vi "Main.vi"(8 "error in (no error)":errorcluster, 11 "ModuleAdmin":refnum<class "ModuleAdmin.lvclass">) -> ()   [LabVIEW 2014, in "ScopeModule.lvlib"]
uses:
  ScopeModule.lvlib
  <userlib>/NIST/ModuleAdminLib/ModuleAdmin/ModuleAdmin.lvclass
  ScopePlugins/ScopePluginBaseClass/ScopePluginsBase.lvclass/ScopePluginsBase.ctl
  PublicAPI/Arguments/Requests/clStopArgument.ctl
  ScopePlugins/ScopePluginBaseClass/ScopePluginsBase.lvclass
  <userlib>/NIST/ModuleAdminLib/ModuleAdmin/ModuleAdmin.lvclass/ModuleAdmin.ctl
  <userlib>/NIST/BaseClasses/BasePlugin_class/BasePlugin.lvclass/BasePlugin.ctl
  ScopePlugins/InfiniiumClass/Typedefs/ExtAcquisition.ctl
  ScopePlugins/TypeDefs/InitOptions.ctl
  <vilib>/Utility/error.llb/DialogType.ctl
  ScopePlugins/ScopePluginBaseClass/Accessors/Read ModuleID.vi
  ScopePlugins/ScopePluginBaseClass/Accessors/Read Acquisition.vi
  ScopePlugins/ScopePluginBaseClass/Accessors/Read Channels.vi
  <userlib>/NIST/ModuleAdminLib/ModuleAdmin/Accessors/Read ShowPanel_.vi
  ScopePlugins/ScopePluginBaseClass/Accessors/Write ModuleID.vi
  <userlib>/NIST/ModuleAdminLib/ModuleAdmin/Accessors/Write ShowPanel_.vi
  <userlib>/NIST/BaseClasses/BasePlugin_class/Accessors/Read PluginIniFilePath.vi
  <userlib>/NIST/ModuleAdminLib/ModuleAdmin/Accessors/Read CloneRegRef.vi
  <vilib>/Utility/error.llb/Error Cluster From Error Code.vi
  <vilib>/ErrorRing/Error Ring.xnode
  <userlib>/NIST/ModuleAdminLib/CloneRegistration/CloneRegistration.lvclass
  <userlib>/NIST/ModuleAdminLib/ModuleAdmin.lvlib
  <userlib>/NIST/BaseClasses/Object_class/BaseObject.lvclass
  ScopePlugins/InfiniiumClass/Infiniium.lvclass
  ScopePlugins/ScopePlugins.lvlib
panel:
  out "error out":errorcluster
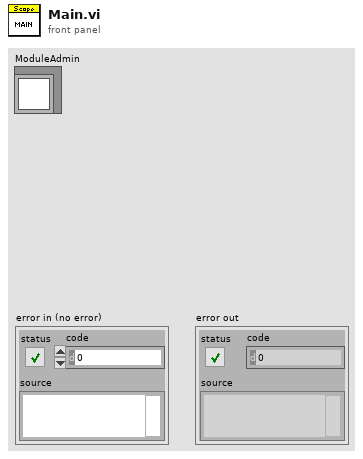
[diagram p1: front panel]
types:
  T1 = typedef "ScopeModule.lvlib/clRequestEvents.ctl" = cluster{"StopRequest":refnum<user-event>, "PathToINI":refnum<user-event>, " LoadPlugin":refnum<user-event>, "ShowPanel":refnum<user-event>, "Abort":refnum<user-event>, "SetAcquisition":refnum<user-event>, "SetChannel":refnum<user-event>, "SetTrigger":refnum<user-event>, "GetAcquisition":refnum<user-event>, "GetChannel":refnum<user-event>, "GetTrigger":refnum<user-event>, "FetchWaveform":refnum<user-event>, "InitAcquisition":refnum<user-event>, "ReadWaveform":refnum<user-event>, "GetHandle":refnum<user-event>, "SetHandle":refnum<user-event>, "GetModel":refnum<user-event>, "SetModel":refnum<user-event>, "ConfigAquisition":refnum<user-event>, "ConfigChannels":refnum<user-event>, "ConfigTrigger":refnum<user-event>, "Initialize":refnum<user-event>, "SetExtAcquisition":refnum<user-event>, "StopAcquisition":refnum<user-event>, "PrefDlg":refnum<user-event>, "Close":refnum<user-event>}
  T2 = typedef "ScopeModule.lvlib/clBroadcastEvents.ctl" = cluster{"DidInit":refnum<user-event>, "StatusUpdate":refnum<user-event>, "ErrorReport":refnum<user-event>, "DidStop":refnum<user-event>, "PathToINI":refnum<user-event>, "Handle":refnum<user-event>, "Model":refnum<user-event>, "Channels":refnum<user-event>, "Acquisition":refnum<user-event>, "Trigger":refnum<user-event>, "ExtAcquisition":refnum<user-event>, "Waveform":refnum<user-event>}
  T3 = typedef "ScopeModule.lvlib/clStopArgument.ctl" = cluster{"Exit via Stop Module Req?":bool, "Wait for Module to stop?":bool, "ModuleAdmin":refnum<class "ModuleAdmin.lvclass">}
  T4 = enum32{"Invalid", "Standard", "Closed", "Hidden", "Minimized", "Maximized"}
  T5 = typedef "ScopePlugins.lvlib/Infiniium.lvclass/ExtAcquisition.ctl" = cluster{"SamplingMode ":enum16{"Real Time", "Equivalent Time", "Segment", "Real Time Peak Detect", "Real Time High Resolution", "Peak Detect Segment", "High Resolution Segment"}, "Interpolation":enum16{"No Interpolation", "sin(x)/x", "linear", "1 Point sin(x)/x", "2 Point sin(x)/x", "4 Point sin(x)/x", "8 Point sin(x)/x", "16 Point sin(x)/x"}, "NumAverages":i32, "EnableAveraging":bool, "Resolution":enum16{"Auto", "Bits 9", "Bits 10", "Bits 11", "Bits 12"}}
  T6 = typedef "ScopePlugins.lvlib/InitOptions.ctl" = cluster{"Reset":bool, "IdQuery":bool}
  T7 = typedef "ScopePlugins.lvlib/Acquisition.ctl" = cluster{"StartTime":dbl, "Type":enum16{"Normal", "PeakDetect", "HighRes", "Envelope", "Average"}, "NumPointsMin":i32, "RecordLength":i32, "SampleRate":dbl, "TimePerRecord":dbl, "SamplingMode ":enum16{"Real Time", "Equivalent Time", "Segment", "Real Time Peak Detect", "Real Time High Resolution", "Peak Detect Segment", "High Resolution Segment"}, "Interpolation":enum16{"No Interpolation", "sin(x)/x", "linear", "1 Point sin(x)/x", "2 Point sin(x)/x", "4 Point sin(x)/x", "8 Point sin(x)/x", "16 Point sin(x)/x"}, "NumAverages":i32, "Resolution":enum16{"Auto", "Bits 9", "Bits 10", "Bits 11", "Bits 12"}, "EnableAveraging":bool, "Continuous":bool}
  T8 = typedef "ScopePlugins.lvlib/Channels.ctl" = cluster{"Count":i32, "ChannelArray":T9[]}
  T9 = typedef "ScopePlugins.lvlib/Channel.ctl" = cluster{"Enabled":bool, "Name":string, "InputImpedance":dbl, "InputFreqMax":dbl, "ProbeAttn":dbl, "Coupling":enum16{"AC", "DC", "GND"}, "Offset":dbl, "Range":dbl, "Handle":string, "Connected":bool}
  T10 = typedef "ScopePlugins.lvlib/Waveform.ctl" = cluster{"initial x":dbl, "x increment":dbl, "waveform array":dbl[]}
  T11 = typedef "DialogType.ctl" = u16
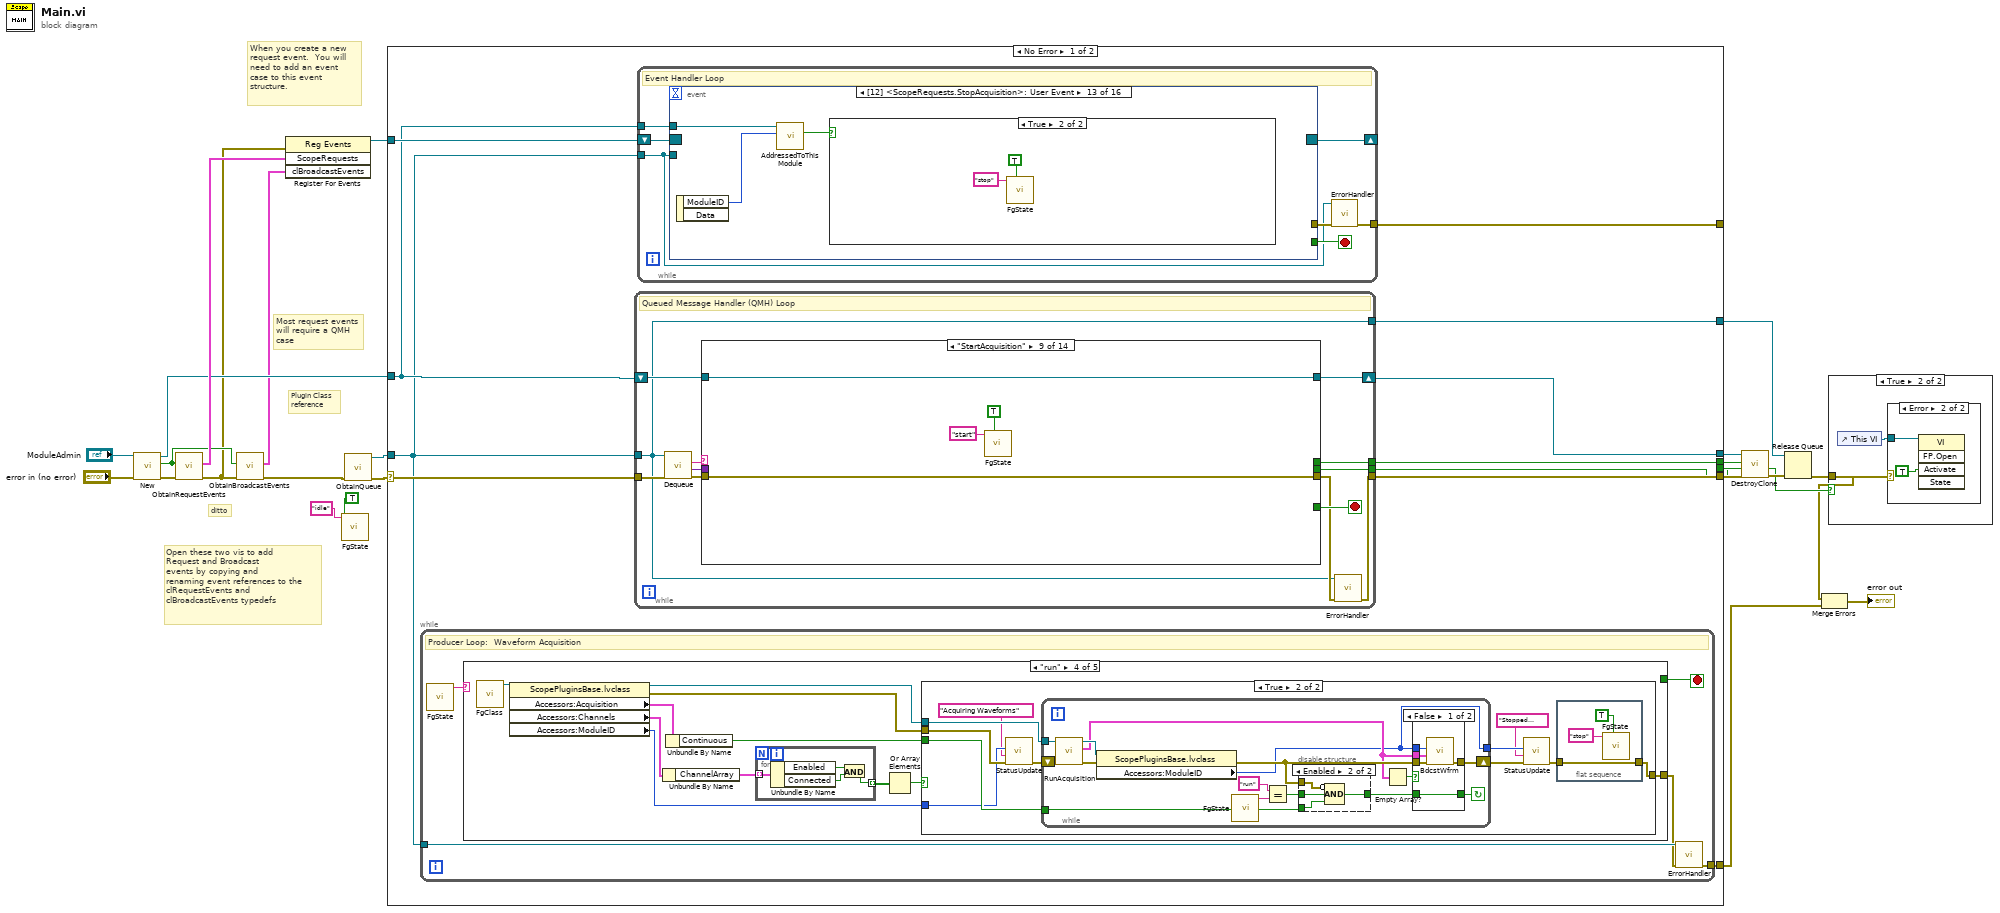
[diagram p0: block diagram]
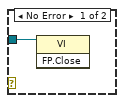
[diagram p3: hidden frame]
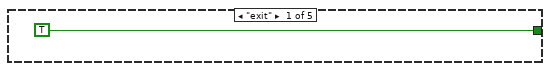
[diagram p4: hidden frame]
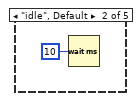
[diagram p5: hidden frame]
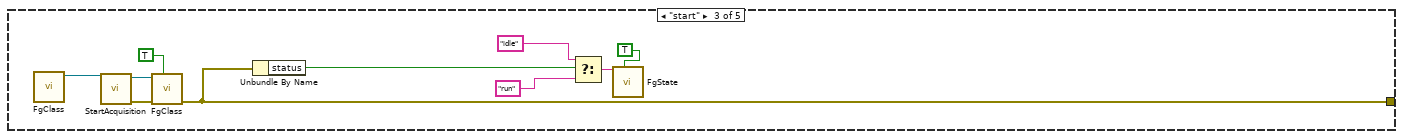
[diagram p6: hidden frame]
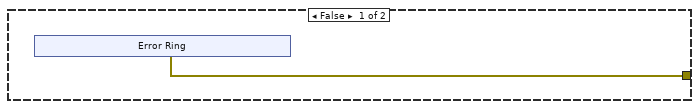
[diagram p7: hidden frame]
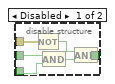
[diagram p8: hidden frame]
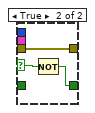
[diagram p9: hidden frame]
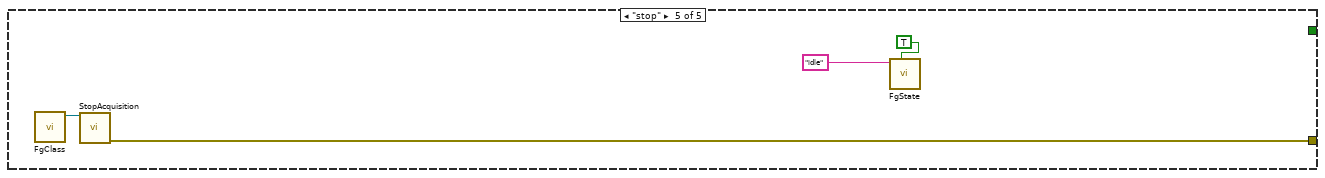
[diagram p10: hidden frame]
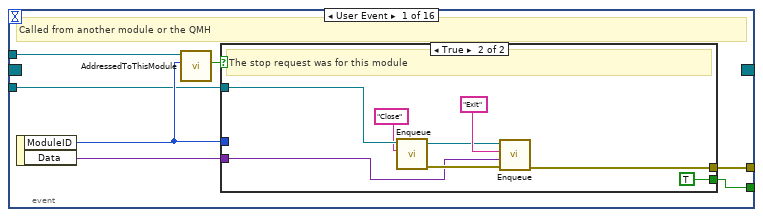
[diagram p11: hidden frame]
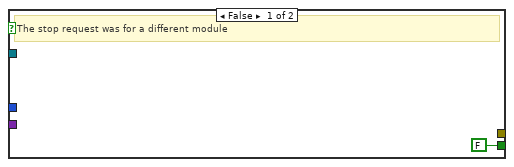
[diagram p12: hidden frame]
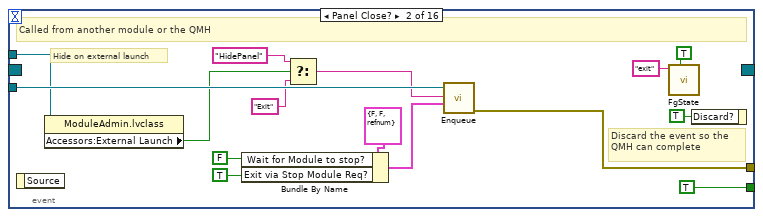
[diagram p13: hidden frame]
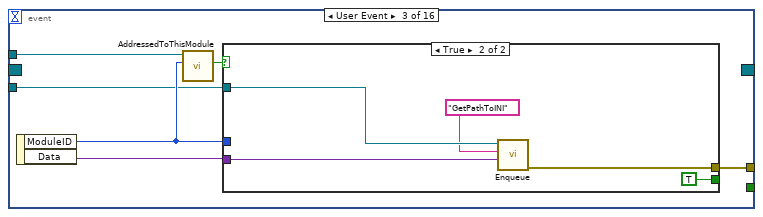
[diagram p14: hidden frame]
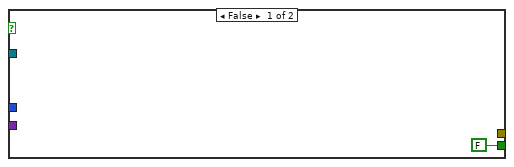
[diagram p15: hidden frame]
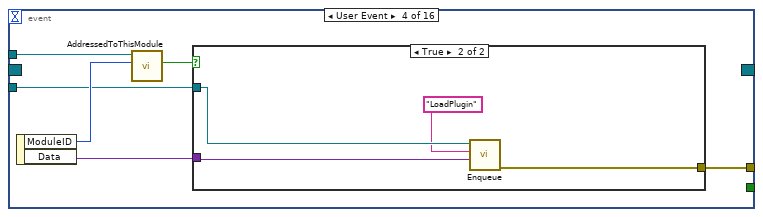
[diagram p16: hidden frame]
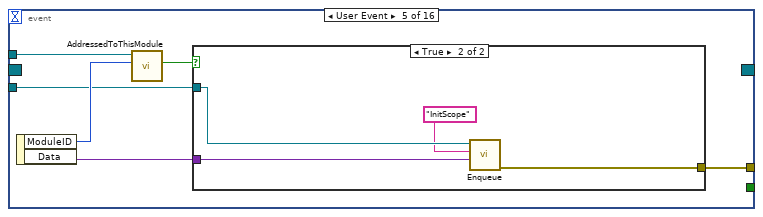
[diagram p18: hidden frame]
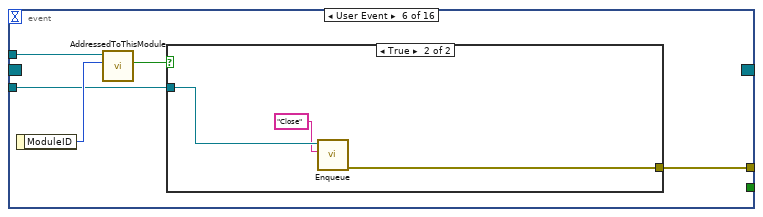
[diagram p20: hidden frame]
diagram:
  # "Plugin Class\nreference"
  # "Open these two vis to add\nRequest and Broadcast \nevents by copying and \nrenaming event references to the \nclRequestEvents and \nclBroadcastEvents typedefs"
  # "ditto"
  # "Most request events\nwill require a QMH\ncase"
  # "When you create a new request event.  You will need to add an event case to this event structure."
  n1 = call <userlib>:"New.vi"("error in (no error)"="error in (no error)", "ModuleAdmin"="ModuleAdmin") -> ("error out"=w22:errorcluster, "First?"=w15:bool, "ModuleAdmin"=w18:refnum<class "ModuleAdmin.lvclass">)  [unwired: 6 in, 1 out]
  n2 = call "ObtainRequestEvents.vi"("error in (no error)"=w22, "CreateNew (F)"=w15) -> ("error out"=w14:errorcluster, "ScopeRequests"=w21:T1)  [unwired: 8 in]
  n3 = call "ObtainBroadcastEvents.vi"("error in (no error)"=w14, "CreateNew? (F)"=w15) -> ("error out"=w16:errorcluster, "clBroadcastEvents"=w13:T2)  [unwired: 8 in]
  n4 = register-events(error in=w14, w21, w13) -> (reference out=w12:refnum<event-registration>)  [unwired: 1 in, 1 out]
  n5 = call "FgState.vi"("Set (F)"=TRUE, "State In"="idle") -> ()  [unwired: 9 in, 1 out]
  n6 = call "ObtainQueue.vi"("error in (no error)"=w16) -> ("error out"=w20:errorcluster, "MessageQueue"=w19:refnum<queue>)  [unwired: 9 in]
  n7 = case shown="No Error" w20 {
    selector: w20 -> [w35 w535]
    tunnel: w19 -> [w26 w531]
    tunnel: w18 -> [w31 w532]
    tunnel: [w34 w533] -> w11
    tunnel: [w33 w531] -> w17
    tunnel: w12 -> [w32 _]
    tunnel: [w30 w530] -> w9
    tunnel: [w29 _] -> w8
    tunnel: [w28 _] -> w7
    tunnel: [w27 _] -> _
    tunnel: [w25 _] -> w1
    frame No Error {
      n8 = while {
        tunnel: w26 -> [w38]
        tunnel: [w36] -> w25
        stop <- w39 stop-if-true
        # "Producer Loop:  Waveform Acquisition"
        n9 = call "FgState.vi"() -> ("State Out"=w40:string)  [unwired: 11 in]
        n10 = case shown="\"run\"" w40 {
          tunnel: [TRUE _ _ _ _] -> w39
          tunnel: [_ _ w48 w61 w120] -> w37
          frame "exit" {
          }
          frame "idle", Default {
            n11 = Wait (ms)(milliseconds to wait=u32 10) -> ()  [unwired: 1 out]
          }
          frame "start" {
            n12 = call "FgClass.vi"() -> ("Class Out"=w51:refnum<class "ScopePluginsBase.lvclass">)  [unwired: 11 in]
            n13 = call-dynamic "StartAcquisition.vi"("ScopePluginsBase in"=w51) -> ("error out"=w48:errorcluster, "ScopePluginsBase out"=w50:refnum<class "ScopePluginsBase.lvclass">)  [unwired: 9 in]
            n14 = call "FgClass.vi"("Set (F)"=TRUE, "Class In"=w50) -> ()  [unwired: 9 in, 1 out]
            n15 = Unbundle By Name(w48) -> ("status"=w46:bool)
            n16 = Select(t="idle" ("State In"), s=w46, f="run") -> (s? t:f=w44:string)
            n17 = call "FgState.vi"("Set (F)"=TRUE, "State In"=w44) -> ()  [unwired: 9 in, 1 out]
          }
          frame "run" {
            n18 = call "FgClass.vi"() -> ("Class Out"=w62:refnum<class "ScopePluginsBase.lvclass">)  [unwired: 11 in]
            n19 = property class="ScopePluginsBase.lvclass"(reference=w62) -> (reference out=w60:refnum<class "ScopePluginsBase.lvclass">, error out=w58:errorcluster, "Accessors:Acquisition"=w53:T7, "Accessors:Channels"=w54:T8, "Accessors:ModuleID"=w52:i32)  [unwired: 1 in]
            n20 = Unbundle By Name(w54) -> ("ChannelArray"=w57:T9[])
            n21 = Unbundle By Name(w53) -> ("Continuous"=w59:bool)
            n22 = for {
              tunnel: w57 -> [w66] mode=indexing
              tunnel: [w63] -> w56 mode=indexing
              n23 = Unbundle By Name(w66) -> ("Enabled"=w65:bool, "Connected"=w64:bool)
              n24 = And(x=w65, y=w64) -> (x .and. y?=w63:bool)
            }
            n25 = Or Array Elements(Boolean array=w56) -> (logical OR=w55:bool)
            n26 = case shown="True" w55 {
              tunnel: [w67 w81] -> w61
              tunnel: w60 -> [_ w83]
              tunnel: w59 -> [_ w82]
              tunnel: w58 -> [_ w80]
              tunnel: w52 -> [_ w78]
              frame False {
                n27 = xnode "Error Ring"() -> ("error out"=w67:errorcluster)
              }
              frame True {
                n28 = call "StatusUpdate.vi"("error in (no error)"=w80, "Status"="Acquiring Waveforms", "ModuleID"=w78) -> ("error out"=w79:errorcluster)  [unwired: 8 in]
                n29 = while {
                  tunnel: w83 -> [w98]
                  tunnel: w82 -> [w97]
                  shift-right: [w95] -> w76
                  shift-left: w79 -> [w96]
                  tunnel: [w84] -> w74
                  stop <- w85 continue-if-true
                  n30 = call-dynamic "RunAcquisition.vi"("error in (no error)"=w96, "ScopePluginsBase in"=w98) -> ("error out"=w90:errorcluster, "Waveforms"=w88:T10[], "ScopePluginsBase out"=w91:refnum<class "ScopePluginsBase.lvclass">)  [unwired: 7 in]
                  n31 = property class="ScopePluginsBase.lvclass"(reference=w91, error in=w90) -> (error out=w89:errorcluster, "Accessors:ModuleID"=w84:i32)  [unwired: 1 out]
                  n32 = call "FgState.vi"() -> ("State Out"=w94:string)  [unwired: 11 in]
                  n33 = Equal?(x="run", y=w94) -> (x = y?=w92:bool)
                  n34 = disable-structure shown="Enabled" {
                    disable-tunnel: w97 -> [w104 w108]
                    disable-tunnel: w92 -> [w103 w106]
                    disable-tunnel: w89 -> [w100 w107]
                    disable-tunnel: [w99 w105] -> w86
                    frame Disabled {
                      n35 = Not(x=w100) -> (.not. x?=w101:bool)
                      n36 = And(x=w103, y=w104) -> (x .and. y?=w102:bool)
                      n37 = And(x=w101, y=w102) -> (x .and. y?=w99:bool)
                    }
                    frame Enabled {
                      n38 = Compound Arithmetic op=AND(invert w107, w106, w108) -> (w105:bool)
                    }
                  }
                  n39 = Empty Array?(array=w88) -> (empty?=w87:bool)
                  n40 = case shown="False" w87 {
                    selector: w87 -> [_ w115]
                    tunnel: [w113 w116] -> w95
                    tunnel: w88 -> [w112 _]
                    tunnel: w84 -> [w111 _]
                    tunnel: w89 -> [w110 w116]
                    tunnel: w86 -> [w109 _]
                    tunnel: [w109 w114] -> w85
                    frame False {
                      n41 = call "BdcstWfrm.vi"("error in (no error)"=w110, "Waveforms"=w112, "ModuleID"=w111) -> ("error out"=w113:errorcluster)  [unwired: 8 in]
                    }
                    frame True {
                      n42 = Not(x=w115) -> (.not. x?=w114:bool)
                    }
                  }
                }
                n43 = call "StatusUpdate.vi"("error in (no error)"=w76, "Status"="Stopped Acquisition", "ModuleID"=w74) -> ("error out"=w75:errorcluster)  [unwired: 8 in]
                n44 = flat-sequence {
                  tunnel: w75 -> [w117]
                  tunnel: [w117] -> w81
                  frame #0 {
                    n45 = call "FgState.vi"("Set (F)"=TRUE, "State In"="stop") -> ()  [unwired: 9 in, 1 out]
                  }
                }
              }
            }
          }
          frame "stop" {
            n46 = call "FgClass.vi"() -> ("Class Out"=w121:refnum<class "ScopePluginsBase.lvclass">)  [unwired: 11 in]
            n47 = call-dynamic "StopAcquisition.vi"("ScopePluginsBase in"=w121) -> ("error out"=w120:errorcluster)  [unwired: 9 in, 1 out]
            n48 = call "FgState.vi"("Set (F)"=TRUE, "State In"="idle") -> ()  [unwired: 9 in, 1 out]
          }
        }
        n49 = call "ErrorHandler.vi"("error in (no error)"=w37, "MessageQueue"=w38) -> ("error out"=w36:errorcluster)  [unwired: 8 in, 1 out]
      }
      n50 = while {
        tunnel: w26 -> [w293]
        tunnel: w35 -> [w302]
        tunnel: [w295] -> w34
        tunnel: [w293] -> w33
        tunnel: [w297] -> w29
        tunnel: [w296] -> w28
        shift-right: [w292] -> w30
        shift-left: w31 -> [w298]
        stop <- w303 stop-if-true
        # "Queued Message Handler (QMH) Loop"
        n51 = call "Dequeue.vi"("error in (no error)"=w302, "MessageQueue"=w293) -> ("error out"=w301:errorcluster, "Message Data"=w299:variant, "Message"=w300:string)  [unwired: 6 in, 1 out]
        n52 = case shown="\"StartAcquisition\"" w300 {
          selector: w300 -> [_ _ _ _ _ _ _ _ _ _ _ _ _ w516]
          tunnel: [_ _ _ _ _ _ _ _ _ _ _ TRUE _ _] -> w303
          tunnel: w298 -> [w326 w342 w351 w357 w404 w419 w432 w446 w453 w465 w474 w490 w504 w519]
          tunnel: [w315 w335 w352 w358 w405 w415 w430 w445 w456 w463 w475 w497 w501 w515] -> w294
          tunnel: w301 -> [_ w345 w349 w367 w409 w418 w433 w447 w456 w471 w483 w489 w505 _]
          tunnel: w299 -> [_ w344 _ w369 w410 _ _ _ _ w472 w482 w493 _ _]
          tunnel: [_ _ _ _ _ _ _ _ _ _ _ w495 _ _] -> w297
          tunnel: [_ _ _ _ _ _ _ _ _ _ _ w494 _ _] -> w296
          tunnel: [w308 w341 w347 w354 w404 w417 w429 w443 w453 w462 w473 w490 w500 w513] -> w292
          frame "Initialize" {
            # "Initialize is always called after ObtainQueue.vi is run"
            n53 = property class="ModuleAdmin.lvclass"(reference=w326) -> (reference out=w313:refnum<class "ModuleAdmin.lvclass">, error out=w323:errorcluster, "Accessors:Module ID"=w304:i32, "Accessors:ShowPanel_"=w311:bool, "Accessors:External Launch"=w310:bool, "Accessors:ModuleName"=w312:string)  [unwired: 1 in]
            n54 = property class="ScopePluginsBase.lvclass"(reference=refnum<class "ScopePluginsBase.lvclass"> refnum ("MyPlugins.lvlib:MyPluginsBase.lvclass"), "Accessors:ModuleID"=w304) -> (reference out=w305:refnum<class "ScopePluginsBase.lvclass">)  [unwired: 1 in, 1 out]
            n55 = Compound Arithmetic op=OR(w311, invert w310) -> (w309:bool)
            n56 = Select(t=T4."Standard" ("Front Panel Window:State"), s=w309, f=T4."Hidden" ("Front Panel Window:State")) -> (s? t:f=w319:T4)
            n57 = call "FgClass.vi"("Set (F)"=TRUE, "Class In"=w305) -> ()  [unwired: 9 in, 1 out]
            n58 = invoke class="VI" method="FP.Open"(error in=w323, "State"=w319) -> (error out=w322:errorcluster)  [unwired: 3 in, 4 out]
            n59 = call <userlib>:"ModuleName.vi"("Name"=w312, "ModuleID"=w304) -> ("ModuleName"=w318:string)  [unwired: 9 in]
            n60 = property class="VI"(error in=w322, "Front Panel.Title"=w318) -> (reference out=w325:refnum<vi>, error out=w324:errorcluster)  [unwired: 1 in]
            n61 = invoke class="VI" method="FP.Center"(reference=w325, error in=w324) -> (error out=w314:errorcluster)  [unwired: 1 in, 2 out]
            n62 = case shown="True" w310 {
              tunnel: [w327 w333] -> w316
              tunnel: [w328 w330] -> w308
              tunnel: w314 -> [w327 w332]
              tunnel: w313 -> [w328 w329]
              frame False {
              }
              frame True {
                n63 = call <userlib>:"WaitOnModuleSync.vi"("error in (no error)"=w332, "ModuleAdmin"=w329) -> ("error out"=w334:errorcluster, "ModuleAdmin"=w331:refnum<class "ModuleAdmin.lvclass">)  [unwired: 8 in]
                n64 = call <userlib>:"WaitOnEventSync.vi"("error in (no error)"=w334, "ModuleAdmin"=w331) -> ("error out"=w333:errorcluster, "ModuleAdmin"=w330:refnum<class "ModuleAdmin.lvclass">)  [unwired: 8 in]
              }
            }
            n65 = call "DidInit.vi"("Init?"=TRUE, "error in (no error)"=w316, "ModuleAdmin"=w308) -> ("error out"=w315:errorcluster)  [unwired: 8 in]
          }
          frame "ShowPanel" {
            n66 = Variant To Data(error in=w345, type=TRUE, Variant=w344) -> (data=w337:bool, error out=w340:errorcluster)
            n67 = Select(t=T4."Standard" ("Front Panel Window:State"), s=w337, f=T4."Hidden" ("Front Panel Window:State")) -> (s? t:f=w336:T4)
            n68 = property class="VI"(error in=w340, "FP.State"=w336) -> (error out=w335:errorcluster)  [unwired: 1 in, 1 out]
            n69 = property class="ModuleAdmin.lvclass"(reference=w342, "Accessors:ShowPanel_"=w337) -> (reference out=w341:refnum<class "ModuleAdmin.lvclass">)  [unwired: 1 in, 1 out]
          }
          frame "GetPathToINI" {
            n70 = call "FgClass.vi"() -> ("Class Out"=w346:refnum<class "ScopePluginsBase.lvclass">)  [unwired: 11 in]
            n71 = property class="ScopePluginsBase.lvclass"(reference=w346, error in=w349) -> (error out=w348:errorcluster, "Accessors:PluginIniFilePath"=w350:path)  [unwired: 1 out]
            n72 = property class="ModuleAdmin.lvclass"(reference=w351) -> (reference out=w347:refnum<class "ModuleAdmin.lvclass">, "Accessors:Module ID"=w353:i32)  [unwired: 1 in, 1 out]
            n73 = call "PathToINIBroadcast.vi"("error in (no error)"=w348, "PathToINI"=w350, "ModuleID"=w353) -> ("error out"=w352:errorcluster)  [unwired: 8 in]
          }
          frame "LoadPlugin" {
            n74 = Variant To Data(error in=w367, type=path "", Variant=w369) -> (data=w355:path, error out=w366:errorcluster)
            n75 = disable-structure shown="Enabled" {
              disable-tunnel: [w372 w373] -> w356
              disable-tunnel: w355 -> [w370 w373]
              frame Disabled {
                n76 = Current VI's Path() -> (path=w371:path)
                n77 = Build Path(base path=w371, name or relative path=w370) -> (appended path=w372:path)
              }
              frame Enabled {
              }
            }
            n78 = call <userlib>:"GetPathToClass.vi"("error in (no error)"=w366, "configuration file path"=w356) -> ("error IO"=w362:errorcluster, "PathToClass"=w365:path)  [unwired: 8 in]
            n79 = Current VI's Path() -> (path=w364:path)
            n80 = Build Path(base path=w364, name or relative path=w365) -> (appended path=w363:path)
            n81 = call <vilib>:"Check if File or Folder Exists.vi"("error in (no error)"=w362, "path"=w363) -> ("error out"=w359:errorcluster, "file or folder exists?"=w361:bool, "dup path"=w360:path)  [unwired: 7 in]
            n82 = case shown="True" w361 {
              tunnel: w360 -> [w376 w392]
              tunnel: w359 -> [_ w400]
              tunnel: [w375 w395] -> w358
              tunnel: w357 -> [w374 w394]
              tunnel: w355 -> [_ w388]
              tunnel: [w374 w391] -> w354
              frame False {
                n83 = Path To String(path=w376) -> (string=w377:string)
                n84 = xnode "Error Ring"("parameter 0"=w377) -> ("error out"=w375:errorcluster)
              }
              frame True {
                n85 = call-dynamic "LoadClassFromFile.vi"("error in (no error)"=w400, "class path"=w392, "reference in"=refnum<class "ScopePluginsBase.lvclass"> refnum ("MyPlugins.lvlib:MyPluginsBase.lvclass")) -> ("error out"=w389:errorcluster, "reference out"=w390:refnum<class "ScopePluginsBase.lvclass">)  [unwired: 7 in]
                n86 = property class="ModuleAdmin.lvclass"(reference=w394) -> (reference out=w391:refnum<class "ModuleAdmin.lvclass">, "Accessors:Module ID"=w393:i32)  [unwired: 1 in, 1 out]
                n87 = call-dynamic "GetDefaultParams.vi"("error in (no error)"=w389, "config file path"=w388, "ScopeBase"=w390) -> ("error out"=w387:errorcluster, "ScopeBase"=w386:refnum<class "ScopePluginsBase.lvclass">)  [unwired: 6 in, 1 out]
                n88 = Path To String(path=w392) -> (string=w397:string)
                n89 = call "FgClass.vi"("Set (F)"=TRUE, "Class In"=w386) -> ()  [unwired: 9 in, 1 out]
                n90 = Format Into String(format string="Plugin %s loaded ", w397) -> (resulting string=w396:string)  [unwired: 2 in, 1 out]
                n91 = call "StatusUpdate.vi"("error in (no error)"=w387, "Status"=w396, "ModuleID"=w393) -> ("error out"=w395:errorcluster)  [unwired: 8 in]
              }
            }
          }
          frame "SetExtAquisition" {
            n92 = Variant To Data(error in=w409, type=T5 {"SamplingMode "=enum."Real Time", "Interpolation"=enum."No Interpolation", "NumAverages"=8, "EnableAveraging"=FALSE, "Resolution"=enum."Auto"} ("ExtAcquisition"), Variant=w410) -> (data=w406:T5, error out=w407:errorcluster)
            n93 = call "FgClass.vi"() -> ("Class Out"=w403:refnum<class "ScopePluginsBase.lvclass">)  [unwired: 11 in]
            n94 = call-dynamic "SetExtAcquisition.vi"("error in (no error)"=w407, "ExtAcquisition"=w406, "ScopePluginsBase in"=w403) -> ("error out"=w405:errorcluster, "ScopePluginsBase out"=w402:refnum<class "ScopePluginsBase.lvclass">)  [unwired: 7 in]
            n95 = call "FgClass.vi"("Set (F)"=TRUE, "Class In"=w402) -> ()  [unwired: 9 in, 1 out]
          }
          frame "ConfigAcquisition" {
            n96 = call "FgClass.vi"() -> ("Class Out"=w413:refnum<class "ScopePluginsBase.lvclass">)  [unwired: 11 in]
            n97 = call-dynamic "ConfigureAcquisition.vi"("error in (no error)"=w418, "ScopePluginsBase in"=w413) -> ("error out"=w416:errorcluster, "ScopePluginsBase out"=w412:refnum<class "ScopePluginsBase.lvclass">)  [unwired: 8 in]
            n98 = call "FgClass.vi"("Set (F)"=TRUE, "Class In"=w412) -> ()  [unwired: 9 in, 1 out]
            n99 = property class="ModuleAdmin.lvclass"(reference=w419) -> (reference out=w417:refnum<class "ModuleAdmin.lvclass">, "Accessors:Module ID"=w414:i32)  [unwired: 1 in, 1 out]
            n100 = case shown="No Error" w416 {
              selector: w416 -> [w423 w424]
              tunnel: [w422 w424] -> w415
              tunnel: w414 -> [w421 _]
              frame No Error {
                n101 = call "StatusUpdate.vi"("error in (no error)"=w423, "Status"="Acquisition Configured", "ModuleID"=w421) -> ("error out"=w422:errorcluster)  [unwired: 8 in]
              }
              frame Error {
              }
            }
          }
          frame "ConfigChannels" {
            n102 = call "FgClass.vi"() -> ("Class Out"=w427:refnum<class "ScopePluginsBase.lvclass">)  [unwired: 11 in]
            n103 = call-dynamic "ConfigureChannels.vi"("error in (no error)"=w433, "ScopePluginsBase in"=w427) -> ("error out"=w431:errorcluster, "ScopePluginsBase out"=w426:refnum<class "ScopePluginsBase.lvclass">)  [unwired: 8 in]
            n104 = call "FgClass.vi"("Set (F)"=TRUE, "Class In"=w426) -> ()  [unwired: 9 in, 1 out]
            n105 = property class="ModuleAdmin.lvclass"(reference=w432) -> (reference out=w429:refnum<class "ModuleAdmin.lvclass">, "Accessors:Module ID"=w428:i32)  [unwired: 1 in, 1 out]
            n106 = case shown="No Error" w431 {
              selector: w431 -> [w437 w438]
              tunnel: [w436 w438] -> w430
              tunnel: w428 -> [w435 _]
              frame No Error {
                n107 = call "StatusUpdate.vi"("error in (no error)"=w437, "Status"="Channels Configured", "ModuleID"=w435) -> ("error out"=w436:errorcluster)  [unwired: 8 in]
              }
              frame Error {
              }
            }
          }
          frame "ConfigTrigger" {
            n108 = call "FgClass.vi"() -> ("Class Out"=w441:refnum<class "ScopePluginsBase.lvclass">)  [unwired: 11 in]
            n109 = call-dynamic "ConfigureTrigger.vi"("error in (no error)"=w447, "ScopePluginsBase in"=w441) -> ("error out"=w444:errorcluster, "ScopePluginsBase out"=w440:refnum<class "ScopePluginsBase.lvclass">)  [unwired: 8 in]
            n110 = call "FgClass.vi"("Set (F)"=TRUE, "Class In"=w440) -> ()  [unwired: 9 in, 1 out]
            n111 = property class="ModuleAdmin.lvclass"(reference=w446) -> (reference out=w443:refnum<class "ModuleAdmin.lvclass">, "Accessors:Module ID"=w442:i32)  [unwired: 1 in, 1 out]
            n112 = case shown="No Error" w444 {
              selector: w444 -> [w451 w452]
              tunnel: [w450 w452] -> w445
              tunnel: w442 -> [w449 _]
              frame No Error {
                n113 = call "StatusUpdate.vi"("error in (no error)"=w451, "Status"="Trigger Configured", "ModuleID"=w449) -> ("error out"=w450:errorcluster)  [unwired: 8 in]
              }
              frame Error {
              }
            }
          }
          frame "StartAcquisition" {
            n114 = call "FgState.vi"("Set (F)"=TRUE, "State In"="start") -> ()  [unwired: 9 in, 1 out]
          }
          frame "InitScope" {
            n115 = Variant To Data(error in=w471, type=T6 {"Reset"=FALSE, "IdQuery"=FALSE} ("InitOptions"), Variant=w472) -> (data=w469:T6, error out=w466:errorcluster)
            n116 = Unbundle By Name(w469) -> ("IdQuery"=w468:bool, "Reset"=w467:bool)
            n117 = call "FgClass.vi"() -> ("Class Out"=w459:refnum<class "ScopePluginsBase.lvclass">)  [unwired: 11 in]
            n118 = call-dynamic "Initialize.vi"("error in (no error)"=w466, "Reset (f)"=w467, "IdQuery (f)"=w468, "ScopePluginsBase in"=w459) -> ("error out"=w464:errorcluster, "ScopePluginsBase out"=w458:refnum<class "ScopePluginsBase.lvclass">)  [unwired: 6 in]
            n119 = call "FgClass.vi"("Set (F)"=TRUE, "Class In"=w458) -> ()  [unwired: 9 in, 1 out]
            n120 = property class="ModuleAdmin.lvclass"(reference=w465) -> (reference out=w462:refnum<class "ModuleAdmin.lvclass">, "Accessors:Module ID"=w461:i32)  [unwired: 1 in, 1 out]
            n121 = call "StatusUpdate.vi"("error in (no error)"=w464, "Status"="O'Scope hardware initialized", "ModuleID"=w461) -> ("error out"=w463:errorcluster)  [unwired: 8 in]
          }
          frame "Error" {
            n122 = property class="ModuleAdmin.lvclass"(reference=w474) -> (reference out=w473:refnum<class "ModuleAdmin.lvclass">, "Accessors:External Launch"=w478:bool, "Accessors:Module ID"=w476:i32)  [unwired: 1 in, 1 out]
            n123 = Variant To Data(error in=w483, type=errorcluster {"status"=FALSE, "code"=0, "source"=""} ("error constant"), Variant=w482) -> (data=w477:errorcluster, error out=w480:errorcluster)
            n124 = call "ReportError.vi"("error in (no error)"=w480, "ErrorReported"=w477, "ModuleID"=w476) -> ("error out"=w479:errorcluster)  [unwired: 8 in]
            n125 = case shown="True" w478 {
              tunnel: w479 -> [w487 w488]
              tunnel: w477 -> [w486 _]
              tunnel: [w485 w488] -> w475
              tunnel: w474 -> [w484 _]
              frame False {
                # "Todo:  Add an event to ask the user\nIf the module should stop or continue"
                # "Stand alone: now, force an exit"
                n126 = call <vilib>:"Simple Error Handler.vi"("error in (no error)"=w486) -> ()  [unwired: 4 in, 5 out]
                n127 = call "StopRequest.vi"("error in (no error)"=w487, "ModuleAdmin"=w484) -> ("error out"=w485:errorcluster)  [unwired: 8 in, 1 out]
              }
              frame True {
                # "Externally launched modules only broadcast the error msg"
              }
            }
          }
          frame "Exit" {
            # "Called by the StopRequest event handler case"
            n128 = control-ref of="This VI"() -> (w496:refnum<vi>)
            n129 = call "FgState.vi"("Set (F)"=TRUE, "State In"="exit") -> ()  [unwired: 9 in, 1 out]
            n130 = call "HandleExit.vi"("error in (no error)"=w489, "VI Refnum"=w496, "StopArgument"=w493, "ModuleAdmin"=w490) -> ("error out"=w497:errorcluster, "Exit via Stop Module Req?"=w494:bool, "WaitForStop?"=w495:bool)  [unwired: 5 in]
          }
          frame "Close" {
            n131 = call "FgClass.vi"() -> ("Class Out"=w507:refnum<class "ScopePluginsBase.lvclass">)  [unwired: 11 in]
            n132 = call-dynamic "Close.vi"("error in (no error)"=w505, "ScopePluginsBase in"=w507) -> ("error out"=w502:errorcluster, "ScopePluginsBase out"=w506:refnum<class "ScopePluginsBase.lvclass">)  [unwired: 8 in]
            n133 = call "FgClass.vi"("Set (F)"=TRUE, "Class In"=w506) -> ()  [unwired: 9 in, 1 out]
            n134 = property class="ModuleAdmin.lvclass"(reference=w504) -> (reference out=w500:refnum<class "ModuleAdmin.lvclass">, "Accessors:Module ID"=w499:i32)  [unwired: 1 in, 1 out]
            n135 = case shown="No Error" w502 {
              selector: w502 -> [w511 w512]
              tunnel: [w510 w512] -> w501
              tunnel: w499 -> [w509 _]
              frame No Error {
                n136 = call "StatusUpdate.vi"("error in (no error)"=w511, "Status"="O'Scope Disconnected", "ModuleID"=w509) -> ("error out"=w510:errorcluster)  [unwired: 8 in]
              }
              frame Error {
              }
            }
          }
          frame Default {
            # "Called only if a message was queued and no QMH case was created"
            n137 = property class="ModuleAdmin.lvclass"(reference=w519) -> (reference out=w513:refnum<class "ModuleAdmin.lvclass">, "Accessors:Module ID"=w518:i32, "Accessors:ModuleName"=w514:string)  [unwired: 1 in, 1 out]
            n138 = call <userlib>:"ModuleName.vi"("Name"=w514, "ModuleID"=w518) -> ("ModuleName"=w517:string)  [unwired: 9 in]
            n139 = xnode "Error Ring"("parameter 0"=w516, "parameter 1"=w517) -> ("error out"=w515:errorcluster)
          }
        }
        n140 = call "ErrorHandler.vi"("error in (no error)"=w294, "MessageQueue"=w293) -> ("error out"=w295:errorcluster)  [unwired: 8 in, 1 out]
      }
      n141 = while {
        tunnel: w26 -> [w124]
        shift-right: [w128] -> _
        shift-left: w32 -> [w129]
        tunnel: w31 -> [w127]
        tunnel: [w125] -> w27
        stop <- w130 stop-if-true
        # "Event Handler Loop"
        n142 = event shown="[12] <ScopeRequests.StopAcquisition>: User Event" {
          selector: w129 -> [_ _ _ _ _ _ _ _ _ _ _ _ _ _ _ _]
          dyn-events: [_ _ _ _ _ _ _ _ _ _ _ _ _ _ _ _] -> w128
          timeout: _ -> [_ _ _ _ _ _ _ _ _ _ _ _ _ _ _ _]
          tunnel: w124 -> [w134 w161 w164 w175 w185 w195 w203 w214 w223 w230 w240 w250 _ w265 w275 w284]
          tunnel: [w133 TRUE _ _ _ _ _ _ _ _ _ _ _ _ _ _] -> w130
          tunnel: w127 -> [w137 w155 w163 w179 w189 w198 w207 w217 w226 w234 w244 w254 w261 w269 w279 w288]
          tunnel: [w132 w159 w162 w176 w186 w194 w204 w212 _ w231 w241 w251 _ w266 w276 w285] -> w126
          event User Event {
            # "Called from another module or the QMH"
            n143 = event-data() -> ("ModuleID"=w135:i32, "Data"=w131:variant)  [unwired: 1 in]
            n144 = call <userlib>:"AddressedToThisModule.vi"("ModuleID"=w135, "ModuleAdmin"=w137) -> ("AddressedToThisInstance?"=w136:bool)  [unwired: 8 in, 1 out]
            n145 = case shown="True" w136 {
              tunnel: w135 -> [_ _]
              tunnel: w134 -> [_ w143]
              tunnel: [FALSE TRUE] -> w133
              tunnel: [_ w145] -> w132
              tunnel: w131 -> [_ w139]
              frame False {
                # "The stop request was for a different module"
              }
              frame True {
                # "The stop request was for this module"
                n146 = call "Enqueue.vi"("Message"="Close", "MessageQueue"=w143) -> ("error out"=w140:errorcluster, "MessageQueue"=w142:refnum<queue>)  [unwired: 8 in]
                n147 = call "Enqueue.vi"("error in (no error)"=w140, "Message Data"=w139, "Message"="Exit", "MessageQueue"=w142) -> ("error out"=w145:errorcluster)  [unwired: 6 in, 1 out]
              }
            }
          }
          event Panel Close? {
            # "Hide on external launch"
            # "Discard the event so the QMH can complete"
            # "Called from another module or the QMH"
            n148 = event-data() -> ()  [unwired: 1 in, 1 out]
            n149 = property class="ModuleAdmin.lvclass"(reference=w155) -> ("Accessors:External Launch"=w150:bool)  [unwired: 1 in, 2 out]
            n150 = Bundle By Name(cluster=T3 {"Exit via Stop Module Req?"=FALSE, "Wait for Module to stop?"=FALSE, "ModuleAdmin"=refnum} ("Stop Argument"), "Wait for Module to stop?"=FALSE, "Exit via Stop Module Req?"=TRUE) -> (w156:T3)
            n151 = Select(t="HidePanel", s=w150, f="Exit" ("Message")) -> (s? t:f=w152:string)
            n152 = call "Enqueue.vi"("Message Data"=w156, "Message"=w152, "MessageQueue"=w161) -> ("error out"=w159:errorcluster)  [unwired: 7 in, 1 out]
            n153 = call "FgState.vi"("Set (F)"=TRUE, "State In"="exit") -> ()  [unwired: 9 in, 1 out]
            n154 = event-data("Discard?"=TRUE) -> ()  [unwired: 1 in, 1 out]
          }
          event User Event {
            n155 = event-data() -> ("ModuleID"=w165:i32, "Data"=w166:variant)  [unwired: 1 in]
            n156 = call <userlib>:"AddressedToThisModule.vi"("ModuleID"=w165, "ModuleAdmin"=w163) -> ("AddressedToThisInstance?"=w167:bool)  [unwired: 8 in, 1 out]
            n157 = case shown="True" w167 {
              tunnel: w165 -> [_ _]
              tunnel: w164 -> [_ w173]
              tunnel: [FALSE TRUE] -> _
              tunnel: [_ w171] -> w162
              tunnel: w166 -> [_ w169]
              frame False {
                # "The stop request was for a different module"
              }
              frame True {
                # "The stop request was for this module"
                n158 = call "Enqueue.vi"("Message Data"=w169, "Message"="GetPathToINI", "MessageQueue"=w173) -> ("error out"=w171:errorcluster)  [unwired: 7 in, 1 out]
              }
            }
          }
          event User Event {
            n159 = event-data() -> ("ModuleID"=w178:i32, "Data"=w174:variant)  [unwired: 1 in]
            n160 = call <userlib>:"AddressedToThisModule.vi"("ModuleID"=w178, "ModuleAdmin"=w179) -> ("AddressedToThisInstance?"=w177:bool)  [unwired: 8 in, 1 out]
            n161 = case shown="True" w177 {
              tunnel: [_ w180] -> w176
              tunnel: w175 -> [_ w183]
              tunnel: w174 -> [_ w181]
              frame False {
              }
              frame True {
                n162 = call "Enqueue.vi"("Message Data"=w181, "Message"="LoadPlugin", "MessageQueue"=w183) -> ("error out"=w180:errorcluster)  [unwired: 7 in, 1 out]
              }
            }
          }
          event User Event {
            n163 = event-data() -> ("ModuleID"=w188:i32, "Data"=w184:variant)  [unwired: 1 in]
            n164 = call <userlib>:"AddressedToThisModule.vi"("ModuleID"=w188, "ModuleAdmin"=w189) -> ("AddressedToThisInstance?"=w187:bool)  [unwired: 8 in, 1 out]
            n165 = case shown="True" w187 {
              tunnel: [_ w190] -> w186
              tunnel: w185 -> [_ w193]
              tunnel: w184 -> [_ w191]
              frame False {
              }
              frame True {
                n166 = call "Enqueue.vi"("Message Data"=w191, "Message"="InitScope", "MessageQueue"=w193) -> ("error out"=w190:errorcluster)  [unwired: 7 in, 1 out]
              }
            }
          }
          event User Event {
            n167 = event-data() -> ("ModuleID"=w197:i32)  [unwired: 1 in]
            n168 = call <userlib>:"AddressedToThisModule.vi"("ModuleID"=w197, "ModuleAdmin"=w198) -> ("AddressedToThisInstance?"=w196:bool)  [unwired: 8 in, 1 out]
            n169 = case shown="True" w196 {
              tunnel: w195 -> [_ w201]
              tunnel: [_ w200] -> w194
              frame False {
              }
              frame True {
                n170 = call "Enqueue.vi"("Message"="Close", "MessageQueue"=w201) -> ("error out"=w200:errorcluster)  [unwired: 8 in, 1 out]
              }
            }
          }
          event User Event {
            n171 = event-data() -> ("ModuleID"=w206:i32, "Data"=w202:variant)  [unwired: 1 in]
            n172 = call <userlib>:"AddressedToThisModule.vi"("ModuleID"=w206, "ModuleAdmin"=w207) -> ("AddressedToThisInstance?"=w205:bool)  [unwired: 8 in, 1 out]
            n173 = case shown="True" w205 {
              tunnel: [_ w208] -> w204
              tunnel: w203 -> [_ w211]
              tunnel: w202 -> [_ w209]
              frame False {
              }
              frame True {
                n174 = call "Enqueue.vi"("Message Data"=w209, "Message"="ShowPanel", "MessageQueue"=w211) -> ("error out"=w208:errorcluster)  [unwired: 7 in, 1 out]
              }
            }
          }
          event User Event {
            n175 = event-data() -> ("ModuleID"=w216:i32, "Data"=w213:variant)  [unwired: 1 in]
            n176 = call <userlib>:"AddressedToThisModule.vi"("ModuleID"=w216, "ModuleAdmin"=w217) -> ("AddressedToThisInstance?"=w215:bool)  [unwired: 8 in, 1 out]
            n177 = case shown="True" w215 {
              tunnel: w214 -> [_ _]
              tunnel: w213 -> [_ _]
              tunnel: [_ w218] -> w212
              frame False {
              }
              frame True {
                n178 = call "FgClass.vi"() -> ("Class Out"=w221:refnum<class "ScopePluginsBase.lvclass">)  [unwired: 11 in]
                n179 = call "ConfigDlg.vi"("ScopePluginsBase in"=w221) -> ("error out"=w218:errorcluster, "ScopePluginsBase out"=w220:refnum<class "ScopePluginsBase.lvclass">)  [unwired: 9 in]
                n180 = call "FgClass.vi"("Set (F)"=TRUE, "Class In"=w220) -> ()  [unwired: 9 in, 1 out]
              }
            }
          }
          event User Event {
            n181 = event-data() -> ("ModuleID"=w225:i32, "Data"=w222:variant)  [unwired: 1 in]
            n182 = call <userlib>:"AddressedToThisModule.vi"("ModuleID"=w225, "ModuleAdmin"=w226) -> ("AddressedToThisInstance?"=w224:bool)  [unwired: 8 in, 1 out]
            n183 = case shown="True" w224 {
              tunnel: w223 -> [_ _]
              tunnel: w222 -> [_ _]
              frame False {
              }
              frame True {
                n184 = call "FgState.vi"("Set (F)"=TRUE, "State In"="stop") -> ()  [unwired: 9 in, 1 out]
              }
            }
          }
          event User Event {
            n185 = event-data() -> ("ModuleID"=w233:i32, "Data"=w229:variant)  [unwired: 1 in]
            n186 = call <userlib>:"AddressedToThisModule.vi"("ModuleID"=w233, "ModuleAdmin"=w234) -> ("AddressedToThisInstance?"=w232:bool)  [unwired: 8 in, 1 out]
            n187 = case shown="True" w232 {
              tunnel: [_ w235] -> w231
              tunnel: w230 -> [_ w238]
              tunnel: w229 -> [_ w236]
              frame False {
              }
              frame True {
                n188 = call "Enqueue.vi"("Message Data"=w236, "Message"="Unhandled Event", "MessageQueue"=w238) -> ("error out"=w235:errorcluster)  [unwired: 7 in, 1 out]
              }
            }
          }
          event User Event {
            n189 = event-data() -> ("ModuleID"=w243:i32, "Data"=w239:variant)  [unwired: 1 in]
            n190 = call <userlib>:"AddressedToThisModule.vi"("ModuleID"=w243, "ModuleAdmin"=w244) -> ("AddressedToThisInstance?"=w242:bool)  [unwired: 8 in, 1 out]
            n191 = case shown="True" w242 {
              tunnel: [_ w245] -> w241
              tunnel: w240 -> [_ w248]
              tunnel: w239 -> [_ w246]
              frame False {
              }
              frame True {
                n192 = call "Enqueue.vi"("Message Data"=w246, "Message"="ConfigAcquisition", "MessageQueue"=w248) -> ("error out"=w245:errorcluster)  [unwired: 7 in, 1 out]
              }
            }
          }
          event User Event {
            n193 = event-data() -> ("ModuleID"=w253:i32, "Data"=w249:variant)  [unwired: 1 in]
            n194 = call <userlib>:"AddressedToThisModule.vi"("ModuleID"=w253, "ModuleAdmin"=w254) -> ("AddressedToThisInstance?"=w252:bool)  [unwired: 8 in, 1 out]
            n195 = case shown="True" w252 {
              tunnel: [_ w255] -> w251
              tunnel: w250 -> [_ w258]
              tunnel: w249 -> [_ w256]
              frame False {
              }
              frame True {
                n196 = call "Enqueue.vi"("Message Data"=w256, "Message"="SetExtAquisition", "MessageQueue"=w258) -> ("error out"=w255:errorcluster)  [unwired: 7 in, 1 out]
              }
            }
          }
          event User Event {
            n197 = event-data() -> ("ModuleID"=w260:i32)  [unwired: 1 in, 1 out]
            n198 = call <userlib>:"AddressedToThisModule.vi"("ModuleID"=w260, "ModuleAdmin"=w261) -> ("AddressedToThisInstance?"=w259:bool)  [unwired: 8 in, 1 out]
            n199 = case shown="True" w259 {
              frame False {
              }
              frame True {
                n200 = call "FgState.vi"("Set (F)"=TRUE, "State In"="stop") -> ()  [unwired: 9 in, 1 out]
              }
            }
          }
          event User Event {
            n201 = event-data() -> ("ModuleID"=w268:i32, "Data"=w264:variant)  [unwired: 1 in]
            n202 = call <userlib>:"AddressedToThisModule.vi"("ModuleID"=w268, "ModuleAdmin"=w269) -> ("AddressedToThisInstance?"=w267:bool)  [unwired: 8 in, 1 out]
            n203 = case shown="True" w267 {
              tunnel: [_ w270] -> w266
              tunnel: w265 -> [_ w273]
              tunnel: w264 -> [_ w271]
              frame False {
              }
              frame True {
                n204 = call "Enqueue.vi"("Message Data"=w271, "Message"="ConfigTrigger", "MessageQueue"=w273) -> ("error out"=w270:errorcluster)  [unwired: 7 in, 1 out]
              }
            }
          }
          event User Event {
            n205 = event-data() -> ("ModuleID"=w278:i32, "Data"=w274:variant)  [unwired: 1 in]
            n206 = call <userlib>:"AddressedToThisModule.vi"("ModuleID"=w278, "ModuleAdmin"=w279) -> ("AddressedToThisInstance?"=w277:bool)  [unwired: 8 in, 1 out]
            n207 = case shown="True" w277 {
              tunnel: [_ w280] -> w276
              tunnel: w275 -> [_ w283]
              tunnel: w274 -> [_ w281]
              frame False {
              }
              frame True {
                n208 = call "Enqueue.vi"("Message Data"=w281, "Message"="ConfigChannels", "MessageQueue"=w283) -> ("error out"=w280:errorcluster)  [unwired: 7 in, 1 out]
              }
            }
          }
          event User Event {
            n209 = event-data() -> ("ModuleID"=w287:i32)  [unwired: 1 in, 1 out]
            n210 = call <userlib>:"AddressedToThisModule.vi"("ModuleID"=w287, "ModuleAdmin"=w288) -> ("AddressedToThisInstance?"=w286:bool)  [unwired: 8 in, 1 out]
            n211 = case shown="True" w286 {
              tunnel: [_ w290] -> w285
              tunnel: w284 -> [_ w289]
              frame False {
              }
              frame True {
                n212 = call "Enqueue.vi"("Message"="StartAcquisition", "MessageQueue"=w289) -> ("error out"=w290:errorcluster)  [unwired: 8 in, 1 out]
              }
            }
          }
        }
        n213 = call "ErrorHandler.vi"("error in (no error)"=w126, "MessageQueue"=w124) -> ("error out"=w125:errorcluster)  [unwired: 8 in, 1 out]
      }
    }
    frame Error {
      n214 = property class="ModuleAdmin.lvclass"(reference=w532) -> (reference out=w530:refnum<class "ModuleAdmin.lvclass">, "Accessors:CloneRegRef"=w529:refnum<data-value>, "Accessors:Module ID"=w528:i32)  [unwired: 1 in, 1 out]
      n215 = call <userlib>:"Remove.vi"("Module ID"=w528, "CloneRegRef"=w529) -> ("error out"=w534:errorcluster)  [unwired: 7 in, 2 out]
      n216 = flat-sequence {
        tunnel: w535 -> [w538]
        tunnel: w534 -> [_]
        tunnel: [w536] -> w533
        frame #0 {
          w537 = T11 2 items=["no dialog", "OK message", "continue or stop message", "OK message + warnings", "continue/stop + warnings"] ("type of dialog (OK msg:1)")
          n217 = call <vilib>:"Simple Error Handler.vi"("type of dialog (OK msg:1)"=w537, "error in (no error)"=w538) -> ("error out"=w536:errorcluster)  [unwired: 3 in, 4 out]
        }
      }
    }
  }
  n218 = call "DestroyClone.vi"("error in (no error)"=w11, "Exit via Stop Module Req?"=w7, "Wait for Module to stop?"=w8, "ModuleAdmin"=w9) -> ("error out"=w10:errorcluster, "External Launch"=w6:bool)  [unwired: 5 in, 1 out]
  n219 = Release Queue(queue=w17, error in (no error)=w10) -> (error out=w5:errorcluster)  [unwired: 1 in, 2 out]
  n220 = Merge Errors(w5, w1) -> (→"error out":errorcluster)
  n221 = case shown="True" w6 {
    tunnel: w5 -> [_ w540]
    frame False {
    }
    frame True {
      n222 = control-ref of="This VI"() -> (w539:refnum<vi>)
      n223 = case shown="Error" w540 {
        tunnel: w539 -> [w541 w542]
        frame No Error {
          n224 = invoke class="VI" method="FP.Close"(reference=w541) -> ()  [unwired: 2 in, 3 out]
        }
        frame Error {
          n225 = invoke class="VI" method="FP.Open"(reference=w542, "Activate"=TRUE ("Activate?")) -> ()  [unwired: 3 in, 5 out]
        }
      }
    }
  }
